vi "picoharp_write_header_legacy.vi"(8 "error in (no error)":errorcluster, 11 "hydraharp in":refnum<class "picoharp.lvclass">) -> (0 "error out":errorcluster, 3 "hydraharp out":refnum<class "picoharp.lvclass">)   [LabVIEW 2015, in "picoharp.lvclass"]
uses:
  picoharp.lvclass
  picoharp.lvclass/picoharp.ctl
  Data Logger Class/data_logger.lvclass
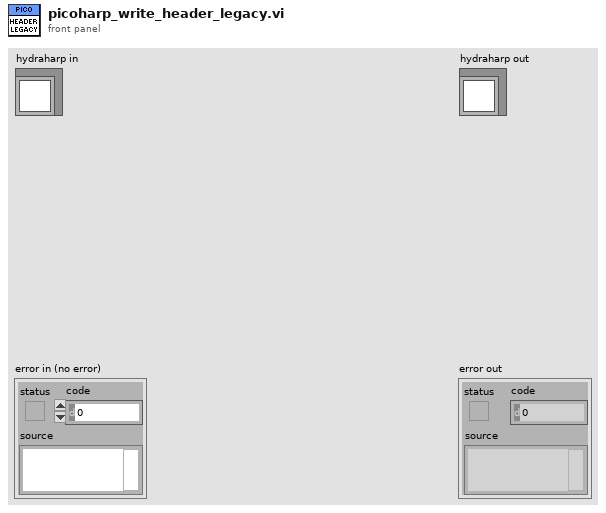
[diagram p1: front panel]
types:
  T1 = typedef "hpanel_hydraharp_settings.ctl" = cluster{"Sync Settings":T2, "CH 1":T4, "CH 2":T4, "CH 3":T4, "CH 4":T4, "binning":i32, "CH 5":T4, "CH 6":T4, "CH 7":T4, "CH 8":T4}
  T2 = typedef "hpanel_sync_settings.ctl" = cluster{"snc_count":i32, "snc_level":i32, "snc_ZeroX":i32, "snc_offs":i32, "sync_div":T3}
  T3 = typedef "hpanel_sync_div.ctl" = enum16{"1", "2", "4", "8"}
  T4 = typedef "hpanel_channel_settings.ctl" = cluster{"ch_counts":i32, "ch_level":i32, "ch_ZeroX":i32, "ch_offs":i32}
  T5 = typedef "hpanel_acq_modes.ctl" = u16
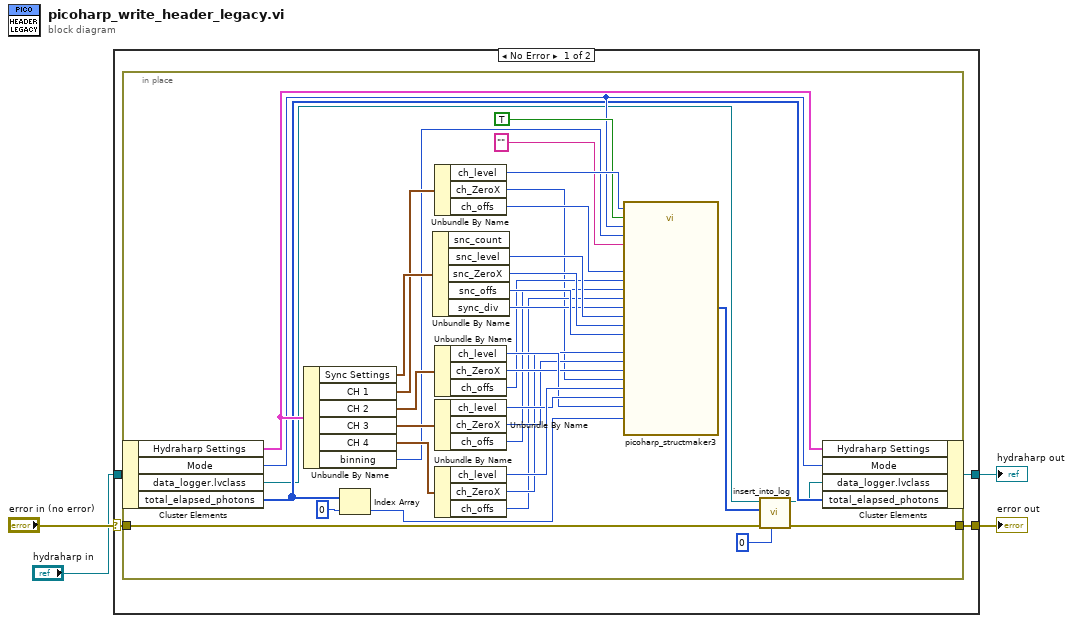
[diagram p0: block diagram]
diagram:
  n1 = case shown="No Error" "error in (no error)" {
    selector: "error in (no error)" -> [w7 w45]
    tunnel: [w5 w45] -> w3
    tunnel: [w6 w44] -> w1
    tunnel: "hydraharp in" -> [w8 w44]
    frame No Error {
      n2 = in-place {
        in-place-border: w7 -> [w11]
        in-place-border: [w10] -> w5
        n3 = in-place-cluster #1(w8) -> ("Hydraharp Settings"=w19:T1, "Mode"=w18:T5, "data_logger.lvclass"=w14:refnum<class "data_logger.lvclass">, "total_elapsed_photons"=w15:i32[])
        n4 = Unbundle By Name(w19) -> ("Sync Settings"=w43:T2, "CH 1"=w41:T4, "CH 2"=w40:T4, "CH 3"=w39:T4, "CH 4"=w38:T4, "binning"=w21:i32)
        n5 = Index Array(array=w15, index=0) -> (element=w16:i32)
        n6 = Unbundle By Name(w43) -> ("snc_level"=w30:i32, "snc_ZeroX"=w31:i32, "snc_offs"=w42:i32, "sync_div"=w29:T3)  [unwired: 1 out]
        n7 = Unbundle By Name(w41) -> ("ch_level"=w23:i32, "ch_ZeroX"=w24:i32, "ch_offs"=w25:i32)
        n8 = Unbundle By Name(w40) -> ("ch_level"=w35:i32, "ch_ZeroX"=w34:i32, "ch_offs"=w26:i32)
        n9 = Unbundle By Name(w39) -> ("ch_level"=w36:i32, "ch_ZeroX"=w33:i32, "ch_offs"=w27:i32)
        n10 = Unbundle By Name(w38) -> ("ch_level"=w37:i32, "ch_ZeroX"=w32:i32, "ch_offs"=w28:i32)
        n11 = call "picoharp_structmaker3.vi"("Channel 3 Zero Cross"=w32, "Channel 2 Zero Cross"=w33, "Channel 1 Zero Cross"=w34, "Channel 0 Zero Cross"=w24, "Channel 3 Discriminator"=w37, "Channel 2 Discriminator"=w36, "Channel 1 Discriminator"=w35, "Channel 0 Discriminator"=w23, "n_records"=w16, "Use user inputs?"=TRUE, "Measurement Mode"=w18, "Binning"=w21, "COMMENT"="", "Sync Offset"=w42, "Sync input Zero Cross Level"=w31, "Sync input Discriminator (mv)"=w30, "Sync Divider"=w29, "Channel 3 Offset"=w28, "Channel  2 Offset"=w27, "Channel 1 offset"=w26, "Channel 0 offset"=w25) -> ("Header in binary"=w12:u8[])  [unwired: 4 in, 2 out]
        n12 = call-dynamic "insert_into_log.vi"("offset_from_bof"=u32 0, "error in (no error)"=w11, "Data"=w12, "data_logger in"=w14) -> ("error out"=w10:errorcluster, "data_logger out"=w13:refnum<class "data_logger.lvclass">)  [unwired: 6 in]
        n13 = in-place-cluster #1("Hydraharp Settings"=w19, "Mode"=w18, "data_logger.lvclass"=w13, "total_elapsed_photons"=w15) -> (w6:refnum<class "picoharp.lvclass">)
      }
    }
    frame Error {
    }
  }
  "error out" <- w3
  "hydraharp out" <- w1
